vi "Encode uint64.vi"(7 "Field Number":i32, 10 "uint64":u64, 11 "Buffer in":u8[](array[numeric]) format="%.0x") -> (3 "Buffer":u8[](array[numeric]) format="%.0x")   [LabVIEW 2020, in "LV-Proto.lvlib"]
uses:
  LV-Proto.lvlib
  Wire Type.ctl
  Wire Encode Varint I32.vi
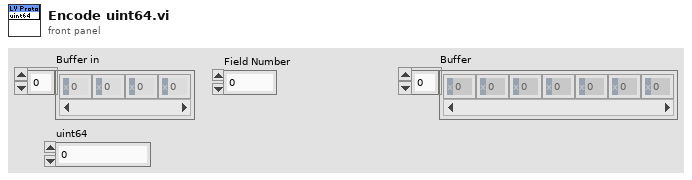
[diagram p1: front panel]
types:
  T1 = typedef "LV-Proto.lvlib/Wire Type.ctl" = enum8{"VARINT", "I64", "LEN", "SGROUP (Deprecated)", "EGROUP (Deprecated)", "I32"}
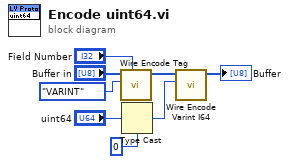
[diagram p0: block diagram]
diagram:
  n1 = call "Wire Encode Tag.vi"("Field Number"="Field Number", "Wire Type"=Wire_Type."VARINT", "Buffer in"="Buffer in") -> ("Buffer"=w4:u8[])  [unwired: 8 in]
  n2 = Type Cast(type=i64 0, x="uint64") -> (*(type *) &x=w2:i64)
  n3 = call "Wire Encode Varint I64.vi"("I64"=w2, "Buffer in"=w4) -> ("Buffer"=→"Buffer":u8[])  [unwired: 9 in]
